vi "FOCUS_V42_H37.vi"(9 "X-pixels":sgl=256.0, 11 "Run":bool) -> (0 "Retrace pixels":sgl, 10 "Pixel Clock (Hz)":sgl)   [LabVIEW 2010] (continued)
            n1850 = Unbundle(w3125) -> ("z-positionstart (um)"=w3187:sgl, "x-positionstart (um)"=w3186:sgl, "y-positionstart (um)"=w3185:sgl, "x-positionstop (um)"=w3184:sgl, "y-positionstop (um)"=w3183:sgl, "z-positionstop (um)"=w3182:sgl, "X-pixels FreeLine"=w3181:sgl, "Y-lines FreeLine"=w3180:sgl, "Pixel Clock (Hz) FreeLine"=w3179:sgl, "Amplitude Factor"=w3171:sgl, "Pixel Clock z (Hz) FreeLine"=w3172:sgl, "phase shift [°]"=w3173:sgl, "Mode selector"=w3156:u16, "Cusp Delay"=w3159:sgl, "Fiberscope\nMode"=w3151:bool, "Pixel Clock (Hz) FScope"=w3149:sgl, "scans to read"=w3148:sgl, "LS X/Y"=w3150:bool, "DataOffset"=w3152:i32, "DataLength"=w3153:i32, "ScanLineLength"=w3154:i32, "ZSinLength"=w3155:i32)
            n1851 = call "ReScaleUDLFOCUS.vi"("ScanLineUDL"=w3146, "x jog"=w3131, "y jog"=w3130, "Rotation"=w3129, "Zoom"=w3128) -> ("ScanLineUDL"=w3145:sgl[][])
            n1852 = Index Array(array=w3145, index (col)=0 ("index (row)")) -> (element=w3178:sgl[])  [unwired: 1 in]
            n1853 = Index Array(array=w3145, index (col)=1 ("index (row)")) -> (element=w3177:sgl[])  [unwired: 1 in]
            n1854 = Bundle("ScanLineUDL"=w3178, "ScanLineUDL"=w3177) -> (w3176:T23)  [unwired: 1 in]
            n1855 = local write "z-positionstart (um)"(w3187) -> ()
            n1856 = local write "x-positionstart (um)"(w3186) -> ()
            n1857 = local write "y-positionstart (um)"(w3185) -> ()
            n1858 = local write "x-positionstop (um)"(w3184) -> ()
            n1859 = local write "y-positionstop (um)"(w3183) -> ()
            n1860 = local write "z-positionstop (um)"(w3182) -> ()
            n1861 = local write "X-pixels FreeLine"(w3181) -> ()
            n1862 = local write "Y-lines FreeLine"(w3180) -> ()
            n1863 = local write "Pixel Clock (Hz) FreeLine"(w3179) -> ()
            n1864 = local write "Amplitude Factor"(w3171) -> ()
            n1865 = local write "Pixel Clock z (Hz) FreeLine"(w3172) -> ()
            n1866 = local write "phase shift [°]"(w3173) -> ()
            n1867 = local write "Mode selector"(w3156) -> ()
            n1868 = local write "Cusp Delay"(w3159) -> ()
            n1869 = local write "Fiberscope\nMode"(w3151) -> ()
            n1870 = local write "Pixel Clock (Hz) FScope"(w3149) -> ()
            n1871 = local write "scans to read"(w3148) -> ()
            n1872 = local write "LS X/Y"(w3150) -> ()
            n1873 = local write "DataOffset"(w3152) -> ()
            n1874 = local write "DataLength"(w3153) -> ()
            n1875 = local write "ScanLineLength"(w3154) -> ()
            n1876 = local write "ZSinLength"(w3155) -> ()
            n1877 = Build Array(w3176) -> (w3175:T24)
            n1878 = local write "XY Graph 1"(w3175) -> ()
            n1879 = local write "XY Graph 2"(w3175) -> ()
            n1880 = local write "Mode selectorFScope"(w3156) -> ()
          }
        }
      }
      frame True {
        w3217 = sgl 1000000.0 ("y")
        w3261 = u8 0 ("Disabled")
        w3283 = 2
        # "Disable & grey/ hide controls"
        n1881 = local read "pixel dwell time [us] FreeLine"() -> (w3206:sgl)
        n1882 = local read "Number of stacks"() -> (w3247:sgl)
        n1883 = local read "Y-lines FreeLine"() -> (w3219:sgl)
        n1884 = local read "pixel dwell time [us]"() -> (w3207:sgl)
        n1885 = local read "frame/line indicator"() -> (w3275:u16)
        n1886 = local read "Number of frames"() -> (w3253:sgl)
        n1887 = local read "X-pixels FreeLine"() -> (w3216:sgl)
        n1888 = Multiply(x=20.0, y=w3216) -> (x*y=w3259:dbl)
        n1889 = Equal?(x=4.0 ("y"), y=w3275) -> (x = y?=w3202:bool)
        n1890 = local read "Y-lines"() -> (w3248:sgl)
        n1891 = local write "IntDevUsed"(FALSE ("IntDevUsed")) -> ()
        n1892 = Multiply(x=w3219, y=w3216) -> (x*y=w3218:sgl)
        n1893 = Greater?(x=w3247, y=sgl 1.0) -> (0:w3245:bool)
        n1894 = Initialize Array(0.0 ("element"), w3259, 3 ("dimension size")) -> (w3262:dbl[][])
        n1895 = property on="Scan format" class="Ring (strict)"("Disabled"=w3283) -> ()  [unwired: 2 in, 2 out]
        n1896 = property on="X-pixels" class="DigNum (strict)"("Disabled"=w3283) -> ()  [unwired: 2 in, 2 out]
        n1897 = property on="Y-lines" class="DigNum (strict)"("Disabled"=w3283) -> ()  [unwired: 2 in, 2 out]
        n1898 = property on="line scan time (ms)" class="DigNum (strict)"("Disabled"=w3283) -> ()  [unwired: 2 in, 2 out]
        n1899 = property on="Measurement cursor\ncheck box" class="Bool (strict)"("Disabled"=w3283) -> ()  [unwired: 2 in, 2 out]
        n1900 = property on="View line check box" class="Bool (strict)"("Disabled"=w3283) -> ()  [unwired: 2 in, 2 out]
        n1901 = property on="Zoom" class="Slide (strict)"("Disabled"=w3261) -> ()  [unwired: 2 in, 2 out]
        n1902 = property on="Rotation" class="Knob (strict)"("Disabled"=w3261) -> ()  [unwired: 2 in, 2 out]
        n1903 = local write "Ready?"(FALSE ("Ready?")) -> ()
        n1904 = Divide(x="Scanner dead time", y=w3206) -> (x/y=w3210:sgl)
        n1905 = local write "XScale"(TRUE ("XScale")) -> ()
        n1906 = property on="RUN button" class="Bool (strict)"("Visible"=FALSE) -> ()  [unwired: 2 in, 2 out]
        n1907 = Greater?(x=w3218, y=w3217) -> (0:w3221:bool)
        n1908 = Divide(x=w3217, y=w3216) -> (x/y=w3215:sgl)
        n1909 = local read "X-pixels"() -> (w3251:sgl)
        n1910 = Or(x=w3202, y=w3200) -> (x .or. y?=w3201:bool)
        n1911 = local read "Mode selectorFScope"() -> (w3239:u16)
        n1912 = case shown="True" w3245 {
          selector: w3245 -> [_ w3296]
          frame False {
          }
          frame True {
            n1913 = local write "Autosave"(w3296) -> ()
          }
        }
        n1914 = Divide(x="Scanner dead time", y=w3207) -> (x/y=w3213:sgl)
        n1915 = Select(t=w3215, s=w3221, f=w3219) -> (s? t:f=w3220:sgl)
        n1916 = local read "Fiberscope\nMode"() -> (w3240:bool)
        n1917 = Add(x=sgl 2.0, y=w3210) -> (x+y=w3209:sgl)
        n1918 = local read "Mode selector"() -> (w3284:u16)
        n1919 = local read "total x pixels"() -> (w3274:sgl)
        n1920 = local read "Intensity"() -> (w3203:sgl)
        n1921 = case shown="False" w3201 {
          tunnel: w3280 -> [w6792 w6794]
          tunnel: [w6790 w6795] -> w3279
          tunnel: w3278 -> [w6793 w6795]
          tunnel: [w6791 w6794] -> w3277
          frame False {
            n1922 = call <vilib>:"DAQmx Start Task.vi"("task/channels in"=w6793, "error in"=w6792) -> ("task out"=w6790:refnum<k21>, "error out"=w6791:errorcluster)  [unwired: 12 in]
          }
          frame True {
          }
        }
        n1923 = Multiply(x=w3248, y=w3253) -> (x*y=w3252:sgl)
        n1924 = Add(x=sgl 2.0, y=w3213) -> (x+y=w3212:sgl)
        n1925 = Round To Nearest(number=w3209) -> (nearest integer value=w3205:sgl)
        n1926 = Initialize Array(u8 0 ("element"), w3251, w3248) -> (w3285:u8[][])
        n1927 = Initialize Array(u8 0 ("element"), w3216, w3220) -> (w3281:u8[][])
        n1928 = Round To Nearest(number=w3212) -> (nearest integer value=w3204:sgl)
        n1929 = while {
          tunnel: w3294 -> [w3441]
          tunnel: w3293 -> [w3440]
          tunnel: w3292 -> [w3439]
          tunnel: [w3438] -> w3291
          tunnel: [w3437] -> w3290
          tunnel: [w3436] -> w3289
          tunnel: [w3386] -> w3288
          tunnel: [w3393] -> w3287
          tunnel: [w3435] -> w3286
          tunnel: w3285 -> [w3434]
          tunnel: w3284 -> [w3433]
          tunnel: w3281 -> [w3432]
          tunnel: w3279 -> [w3431]
          tunnel: w3277 -> [w3430]
          tunnel: w3274 -> [w3429]
          tunnel: [w3428] -> w3272
          tunnel: [w3427] -> w3271
          tunnel: [w3425] -> w3269
          tunnel: w3267 -> [w3424]
          tunnel: w3266 -> [w3423]
          tunnel: w3262 -> [w3419]
          tunnel: w3216 -> [w3418]
          tunnel: w3243 -> [w3406]
          tunnel: w3244 -> [w3405]
          tunnel: w3258 -> [w3408]
          tunnel: w3257 -> [w3407]
          tunnel: [w3383] -> w3256
          tunnel: [w3397] -> w3255
          tunnel: w3242 -> [w3381]
          tunnel: w3241 -> [w3380]
          tunnel: w3254 -> [w3417]
          tunnel: w3252 -> [w3416]
          tunnel: w3251 -> [w3415]
          tunnel: [w3414] -> w3250
          tunnel: [w3413] -> w3249
          tunnel: w3248 -> [w3412]
          tunnel: w3220 -> [w3411]
          tunnel: w3240 -> [w3373]
          tunnel: w3239 -> [w3372]
          tunnel: w3238 -> [w3371]
          tunnel: w3237 -> [w3370]
          tunnel: w3236 -> [w3369]
          tunnel: w3235 -> [w3368]
          tunnel: w3234 -> [w3367]
          tunnel: [w3366] -> w3233
          tunnel: [w3365] -> w3232
          tunnel: w3231 -> [w3364]
          tunnel: [w3351] -> w3230
          tunnel: w3229 -> [w3341]
          tunnel: w3228 -> [w3340]
          tunnel: [w3339] -> w3227
          tunnel: [w3336] -> w3226
          tunnel: [w3332] -> w3225
          tunnel: [w3331] -> w3224
          tunnel: w3223 -> [w3330]
          tunnel: w3222 -> [w3329]
          tunnel: w3204 -> [w3308]
          tunnel: w3205 -> [w3307]
          tunnel: w3203 -> [w3305]
          tunnel: w3200 -> [w3298]
          i -> [w3402]
          stop <- w3399 stop-if-true
          n1930 = local read "Trigger?"() -> (w3376:bool)
          n1931 = local write "Intensity"(w3305) -> ()
          n1932 = flat-sequence {
            tunnel: w3405 -> [w6664]
            tunnel: w3406 -> [w6663]
            tunnel: [w6662] -> w3303
            tunnel: [w6661] -> w3304
            frame #0 {
              n1933 = call <vilib>:"DAQmx Start Task.vi"("task/channels in"=w6664, "error in"=w6663) -> ("task out"=w6661:refnum<k21>, "error out"=w6662:errorcluster)  [unwired: 12 in]
            }
          }
          n1934 = property class="DAQmx Write"(reference=w3304, error in=w3303) -> ("Status:Total Samples Per Channel Generated"=w3302:dbl)  [unwired: 2 out]
          n1935 = case shown="True" w3376 {
            tunnel: w3408 -> [w6630 w6639]
            tunnel: w3407 -> [w6629 w6638]
            tunnel: [w6628 w6636] -> w3389
            tunnel: [w6627 w6637] -> w3388
            tunnel: w3303 -> [w6624 w6633]
            tunnel: w3304 -> [w6625 w6635]
            tunnel: [w6625 w6634] -> w3375
            tunnel: [w6624 w6632] -> w3374
            tunnel: w3302 -> [_ w6631]
            frame False {
              w6626 = TRUE ("data")
              # "open shutter before\ngathering data"
              n1936 = call-poly <vilib>:"DAQmx Write (Digital Bool 1Line 1Point).vi"("task/channels in"=w6630, "data"=w6626, "error in"=w6629) -> ("task out"=w6627:refnum<k21>, "error out"=w6628:errorcluster)  [unwired: 10 in, 1 out]
              "Shutter open" <- w6626
            }
            frame True {
              n1937 = while {
                tunnel: w6639 -> [w6653]
                tunnel: w6638 -> [w6652]
                tunnel: [w6651] -> w6637
                tunnel: [w6647] -> w6636
                tunnel: w6635 -> [w6650]
                tunnel: [w6649] -> w6634
                tunnel: w6633 -> [w6648]
                tunnel: [w6646] -> w6632
                tunnel: w6631 -> [w6640]
                stop <- w6643 stop-if-true
                n1938 = property class="DAQmx Write"(reference=w6650, error in=w6648) -> (reference out=w6649:refnum<k21>, error out=w6646:errorcluster, "Status:Total Samples Per Channel Generated"=w6641:dbl)
                n1939 = Unbundle By Name(w6646) -> ("status"=w6644:bool)
                n1940 = Not Equal?(x=w6641, y=w6640) -> (x != y?=w6642:bool)
                n1941 = case shown="True" w6642 {
                  tunnel: w6653 -> [w6655 w6659]
                  tunnel: w6652 -> [w6654 w6658]
                  tunnel: [w6655 w6657] -> w6651
                  tunnel: [w6654 w6656] -> w6647
                  frame False {
                  }
                  frame True {
                    w6660 = TRUE ("data")
                    n1942 = local write "Shutter open"(w6660) -> ()
                    n1943 = call-poly <vilib>:"DAQmx Write (Digital Bool 1Line 1Point).vi"("task/channels in"=w6659, "data"=w6660, "error in"=w6658) -> ("task out"=w6657:refnum<k21>, "error out"=w6656:errorcluster)  [unwired: 10 in, 1 out]
                  }
                }
                n1944 = Unbundle By Name(w6647) -> ("status"=w6645:bool)
                n1945 = Compound Arithmetic op=OR(w6642, w6645, w6644) -> (w6643:bool)
              }
            }
          }
          n1946 = local read "Pixel Clock (Hz) FScope"() -> (w3360:sgl)
          n1947 = Initialize Array(u8 0 ("element"), 768 ("dimension size")) -> (w3309:u8[])
          n1948 = local read "Scan mode"() -> (w3306:u16)
          n1949 = local write "Save?"(FALSE ("Save?")) -> ()
          n1950 = Reciprocal(x=w3360) -> (1/x=w3359:sgl)
          n1951 = local read "frame/line indicator"() -> (w3410:u16)
          n1952 = local read "ScanLineFreeLine"() -> (w3321:sgl[][])
          n1953 = Decrement(x="Number of stacks") -> (x-1=w3403:sgl)
          n1954 = flat-sequence {
            tunnel: w3426 -> [w6767]
            tunnel: [w6767] -> w3425
            tunnel: w3352 -> [_]
            tunnel: w3333 -> [_]
            tunnel: [w6729] -> w3323
            frame #0 {
              w6741 = "filename000000"  # name
              n1955 = local read "Pixel Clock z (Hz) FreeLine"() -> (w6738:sgl)
              n1956 = local read "Pixel Clock (Hz) FreeLine"() -> (w6757:sgl)
              n1957 = local read "Pixel Clock (Hz) FScope"() -> (w6732:sgl)
              n1958 = local read "x-positionstart (um)"() -> (w6765:sgl)
              n1959 = local read "y-positionstart (um)"() -> (w6764:sgl)
              n1960 = local read "z-positionstart (um)"() -> (w6766:sgl)
              n1961 = local read "x-positionstop (um)"() -> (w6763:sgl)
              n1962 = local read "y-positionstop (um)"() -> (w6761:sgl)
              n1963 = local read "z-positionstop (um)"() -> (w6762:sgl)
              n1964 = local read "ScanLineLength"() -> (w6754:i32)
              n1965 = local read "X-pixels FreeLine"() -> (w6759:sgl)
              n1966 = local read "Amplitude Factor"() -> (w6737:sgl)
              n1967 = local read "Fiberscope\nMode"() -> (w6733:bool)
              n1968 = local read "Y-lines FreeLine"() -> (w6758:sgl)
              n1969 = local read "DataLength"() -> (w6755:i32)
              n1970 = local read "DataOffset"() -> (w6740:i32)
              n1971 = local read "phase shift [°]"() -> (w6739:sgl)
              n1972 = local read "ZSinLength"() -> (w6753:i32)
              n1973 = local read "Mode selector"() -> (w6756:u16)
              n1974 = local read "scans to read"() -> (w6731:sgl)
              n1975 = local read "Cusp Delay"() -> (w6736:sgl)
              n1976 = local read "LS X/Y"() -> (w6730:bool)
              n1977 = Bundle("z-positionstart (um)"=w6766, "x-positionstart (um)"=w6765, "y-positionstart (um)"=w6764, "x-positionstop (um)"=w6763, "y-positionstop (um)"=w6761, "z-positionstop (um)"=w6762, "X-pixels FreeLine"=w6759, "Y-lines FreeLine"=w6758, "Pixel Clock (Hz) FreeLine"=w6757, "Amplitude Factor"=w6737, "Pixel Clock z (Hz) FreeLine"=w6738, "phase shift [°]"=w6739, "Mode selector"=w6756, "Cusp Delay"=w6736, "Fiberscope\nMode"=w6733, "Pixel Clock (Hz) FScope"=w6732, "scans to read"=w6731, "LS X/Y"=w6730, "DataOffset"=w6740, "DataLength"=w6755, "ScanLineLength"=w6754, "ZSinLength"=w6753) -> (w6760:T22)  [unwired: 1 in]
              n1978 = local read "ScanSignals"() -> (w6744:dbl[][])
              n1979 = Index Array(array=w6744, index (col)=0 ("disabled index (col)")) -> (element=w6747:dbl[])  [unwired: 1 in]
              n1980 = Index Array(array=w6744, index (col)=1 ("disabled index (col)")) -> (element=w6752:dbl[])  [unwired: 1 in]
              n1981 = local read "Retrace pixels"() -> (w6775:sgl)
              n1982 = local read "line scan time (ms)"() -> (w6776:sgl)
              n1983 = Array Max & Min(array=w6747) -> (max value=w6748:dbl, min value=w6749:dbl)  [unwired: 2 out]
              n1984 = local read "Scan Block Length"() -> (w6782:sgl)
              n1985 = local read "Number of frames"() -> (w6778:sgl)
              n1986 = Array Max & Min(array=w6752) -> (max value=w6750:dbl, min value=w6751:dbl)  [unwired: 2 out]
              n1987 = local read "Number of stacks"() -> (w6735:sgl)
              n1988 = local read "Program Version"() -> (w6789:u16)
              n1989 = local read "Time interval [s]"() -> (w6734:sgl)
              n1990 = local read "Pixel Clock (Hz)"() -> (w6781:sgl)
              n1991 = local read "IntDevUsed"() -> (w6784:bool)
              n1992 = local read "x-step (um)"() -> (w6773:sgl)
              n1993 = local read "y-step (um)"() -> (w6772:sgl)
              n1994 = local read "z-step (um)"() -> (w6774:sgl)
              n1995 = Subtract(x=w6748, y=w6749) -> (x-y=w6743:dbl)
              n1996 = Subtract(x=w6750, y=w6751) -> (x-y=w6742:dbl)
              n1997 = local read "Averaging"() -> (w6777:u16)
              n1998 = local read "Intensity"() -> (w6783:sgl)
              n1999 = local read "Rotation"() -> (w6769:sgl)
              n2000 = local read "X-pixels"() -> (w6780:sgl)
              n2001 = local read "Y-lines"() -> (w6779:sgl)
              n2002 = local read "Zoom"() -> (w6768:sgl)
              n2003 = local read "x jog"() -> (w6771:sgl)
              n2004 = local read "y jog"() -> (w6770:sgl)
              n2005 = local read "Date"() -> (w6787:string)
              n2006 = local read "start"() -> (w6786:u32)
              n2007 = local read "Time"() -> (w6788:string)
              n2008 = local read "stop"() -> (w6785:u32)
              n2009 = Bundle("Program Version"=w6789, "name"=w6741, "Time"=w6788, "Date"=w6787, "start"=w6786, "stop"=w6785, "IntDevUsed"=w6784, "Intensity"=w6783, "Scan Block Length"=w6782, "Pixel Clock (Hz)"=w6781, "X-pixels"=w6780, "Y-lines"=w6779, "Number of frames"=w6778, "Averaging"=w6777, "line scan time (ms)"=w6776, "Retrace pixels"=w6775, "z-step (um)"=w6774, "x-step (um)"=w6773, "y-step (um)"=w6772, w6743, w6742, "x jog"=w6771, "y jog"=w6770, "Rotation"=w6769, "Zoom"=w6768, "Number of stacks"=w6735, "Time interval [s]"=w6734, w6760) -> (w6728:T21)  [unwired: 1 in]
              n2010 = call "HeadertestFOCUS.vi"("HeaderCluster"=w6728) -> ("Header"=w6729:u8[])
              "Header" <- w6729
            }
          }
          n2011 = Equal?(x=w3410, y=u16 1) -> (x = y?=w3400:bool)
          n2012 = local read "Parameters"() -> (w3382:T2)
          n2013 = case shown="False" w3373 {
            tunnel: w3441 -> [w3517 w6050]
            tunnel: w3440 -> [w3516 w6049]
            tunnel: w3439 -> [w3515 w6048]
            tunnel: [w3514 w6022] -> w3438
            tunnel: [w3513 w6023] -> w3437
            tunnel: [w3512 w6024] -> w3436
            tunnel: [w3511 w6027] -> w3435
            tunnel: w3434 -> [w3510 w6019]
            tunnel: w3433 -> [w3509 _]
            tunnel: w3432 -> [w3508 _]
            tunnel: w3431 -> [w3507 w6039]
            tunnel: w3430 -> [w3506 w6038]
            tunnel: w3429 -> [w3505 _]
            tunnel: [w3504 w6020] -> w3428
            tunnel: [w3503 w6021] -> w3427
            tunnel: [w3502 w6028] -> w3426
            tunnel: w3424 -> [w3501 w6043]
            tunnel: w3423 -> [w3500 w6042]
            tunnel: [w3499 w6029] -> w3422
            tunnel: [w3498 w6030] -> w3421
            tunnel: [w3497 w6031] -> w3420
            tunnel: w3419 -> [w3496 _]
            tunnel: w3418 -> [w3495 _]
            tunnel: w3417 -> [w3494 w6037]
            tunnel: w3416 -> [w3493 _]
            tunnel: w3415 -> [w3492 w6010]
            tunnel: [w3491 w6035] -> w3414
            tunnel: [w3490 w6034] -> w3413
            tunnel: w3412 -> [w3489 w6006]
            tunnel: w3411 -> [w3488 _]
            tunnel: [w3487 w6036] -> w3343
            tunnel: [w3486 w6033] -> w3396
            tunnel: [w3485 w6032] -> w3395
            tunnel: [w3484 w6026] -> w3394
            tunnel: w3389 -> [w3483 w6040]
            tunnel: w3388 -> [w3482 w6041]
            tunnel: [w3481 w6025] -> w3387
            tunnel: w3382 -> [w3480 _]
            tunnel: w3381 -> [w3479 w6047]
            tunnel: w3380 -> [w3478 w6046]
            tunnel: [w3477 w6009] -> w3377
            tunnel: w3375 -> [w3476 w6045]
            tunnel: w3374 -> [w3475 w6044]
            tunnel: w3372 -> [_ w6051]
            tunnel: w3371 -> [_ w6018]
            tunnel: w3370 -> [_ w6017]
            tunnel: w3369 -> [_ w6016]
            tunnel: w3368 -> [w3473 w6015]
            tunnel: w3367 -> [w3474 w6014]
            tunnel: [w3473 w6013] -> w3366
            tunnel: [w3474 w6012] -> w3365
            tunnel: w3359 -> [_ w6007]
            tunnel: [w3472 w6002] -> w3339
            tunnel: [w3471 w6001] -> w3336
            tunnel: w3341 -> [w3470 _]
            tunnel: w3340 -> [w3469 _]
            tunnel: [w3468 w6000] -> w3332
            tunnel: [w3467 w5999] -> w3331
            tunnel: w3330 -> [w3466 w6000]
            tunnel: w3329 -> [w3465 w5999]
            tunnel: w3309 -> [w3464 _]
            tunnel: w3308 -> [w3463 _]
            tunnel: w3307 -> [w3462 _]
            tunnel: w3306 -> [w3461 _]
            tunnel: w3298 -> [w3460 _]
            tunnel: "Channel selector" -> [w3459 _]
            frame False {
              n2014 = case shown="0, Default" w3509 {
                tunnel: w3475 -> [w3617 w4234 w4719 w5022 w5261 w5724]
                tunnel: w3476 -> [w3640 w4235 w4743 w5023 w5260 w5726]
                tunnel: w3517 -> [w3639 w4242 w4740 w5031 w5297 w5796]
                tunnel: w3516 -> [w3638 w4243 w4741 w5030 w5298 w5795]
                tunnel: w3515 -> [w3637 w4244 w4742 w5029 w5299 w5794]
                tunnel: [w3636 w4242 w4740 w5031 w5297 w5796] -> w3514
                tunnel: [w3635 w4243 w4741 w5030 w5298 w5795] -> w3513
                tunnel: [w3634 w4244 w4742 w5029 w5299 w5794] -> w3512
                tunnel: [w3628 w4233 w4743 w5021 w5262 w5725] -> w3481
                tunnel: [w3618 w4232 w4719 w5020 w5271 w5723] -> w3484
                tunnel: [w3629 w4247 w4737 w5026 w5265 w5791] -> w3511
                tunnel: [w3613 w4238 w4731 w5009 w5264 w5787] -> w3502
                tunnel: w3501 -> [w3633 w4246 w4738 w5027 w5301 w5792]
                tunnel: w3500 -> [w3616 w4241 w4734 w5012 w5288 w5786]
                tunnel: w3510 -> [w3631 w4220 _ _ w5300 _]
                tunnel: w3505 -> [w3632 w4245 w4739 _ w5290 _]
                tunnel: w3508 -> [_ _ _ w5028 _ w5793]
                tunnel: w3495 -> [_ _ _ w4989 _ w5749]
                tunnel: w3507 -> [w3604 w4217 w4736 w5024 w5281 w5789]
                tunnel: w3506 -> [w3603 w4216 w4720 w4987 w5280 w5760]
                tunnel: [w3601 w4214 w4720 w4987 w5278 w5760] -> w3490
                tunnel: [w3602 w4215 w4736 w5024 w5279 w5789] -> w3491
                tunnel: w3479 -> [w3577 w4228 w4723 w5016 w5263 w5782]
                tunnel: w3478 -> [w3576 w4226 w4722 w5015 w5258 w5781]
                tunnel: [w3577 w4227 w4723 w5014 w5263 w5779] -> w3504
                tunnel: [w3576 w4225 w4722 w5013 w5258 w5780] -> w3503
                tunnel: [_ 0 ("DataLength") 0 ("DataLength") 0 ("DataLength") 0 ("DataLength") _] -> w3499
                tunnel: [_ 0 ("DataLength") 0 ("DataLength") 0 ("DataLength") 0 ("DataLength") _] -> w3498
                tunnel: [_ 768 ("DataLength") 768 ("DataLength") 768 ("DataLength") 768 ("DataLength") 768 ("DataLength")] -> w3497
                tunnel: w3496 -> [_ _ _ w5003 _ w5775]
                tunnel: w3482 -> [w3612 w4224 w4727 w4993 w5277 w5765]
                tunnel: w3483 -> [w3611 w4223 w4726 w4992 w5276 w5764]
                tunnel: [w3610 w4213 w4725 w4991 w5275 w5762] -> w3486
                tunnel: [w3609 w4222 w4724 w4990 w5274 w5763] -> w3485
                tunnel: w3494 -> [w3591 w4177 w4709 w4985 w5250 w5756]
                tunnel: [w3589 w4221 w4709 w4985 w5250 w5756] -> w3487
                tunnel: w3493 -> [_ w4218 w4714 _ w5273 _]
                tunnel: w3492 -> [_ w4219 w4713 _ w5272 _]
                tunnel: w3489 -> [w3545 _ _ _ _ _]
                tunnel: w3488 -> [_ _ _ _ _ w5735]
                tunnel: w3480 -> [w3579 _ _ _ _ _]
                tunnel: [_ w4212 w4721 w4988 w5259 w5761] -> w3477
                tunnel: [w3562 w4207 w4711 w4981 w5252 w5755] -> w3472
                tunnel: [w3561 w4206 w4710 w4980 w5251 w5754] -> w3471
                tunnel: w3470 -> [_ _ _ w4981 _ w5755]
                tunnel: w3469 -> [_ _ _ w4980 _ w5754]
                tunnel: [w3560 w4205 w4708 w4979 w5249 w5752] -> w3468
                tunnel: [w3559 w4204 w4707 w4978 w5248 w5753] -> w3467
                tunnel: w3466 -> [w3560 w4205 w4708 _ w5249 _]
                tunnel: w3465 -> [w3559 w4204 w4707 _ w5248 _]
                tunnel: w3464 -> [w3526 w4190 w4693 w4963 w5234 w5731]
                tunnel: w3463 -> [w3553 w4189 w4692 _ w5233 _]
                tunnel: w3462 -> [_ _ _ w4962 _ w5712]
                tunnel: w3461 -> [w3552 w4178 w4691 _ w5232 _]
                tunnel: w3460 -> [w3538 _ _ _ _ _]
                tunnel: w3459 -> [w3523 w4169 w4690 w4961 w5229 w5711]
                frame 0, Default {
                  w3581 = FALSE ("button 1")
                  n2015 = local read "Position piezo [µm]"() -> (w3549:sgl)
                  n2016 = property on="Property Node" class="VI"() -> ("VI Path"=w3531:path)  [unwired: 2 in, 2 out]
                  n2017 = local read "[µm] per pixel at zoom 1"() -> (w3546:sgl)
                  n2018 = Strip Path(path=w3531) -> (stripped path=w3532:path)  [unwired: 1 out]
                  n2019 = flat-sequence {
                    tunnel: w3616 -> [w3649]
                    tunnel: [w3649] -> w3615
                    frame #0 {
                      n2020 = Tick Count (ms)() -> (millisecond timer value=w3650:u32)
                      n2021 = local write "Parameters"(T2."Offset Rotation" ("Parameters")) -> ()
                      n2022 = local write "start"(w3650) -> ()
                    }
                  }
                  n2023 = local read "scattering length [µm]"() -> (w3540:sgl)
                  n2024 = case shown="True" "FocusModeSelector" {
                    tunnel: [w3641 w3647] -> w3619
                    tunnel: [w3642 w3646] -> w3578
                    frame True {
                      n2025 = local read "Scan Block Length"() -> (w3642:sgl)
                      n2026 = Multiply(x=w3642, y=u32 1) -> (x*y=w3643:sgl)
                      n2027 = To Long Integer(number=w3643) -> (32bit integer=w3641:i32)
                    }
                    frame False {
                      n2028 = local read "Scan Block Length"() -> (w3646:sgl)
                      n2029 = To Long Integer(number=0 ("y")) -> (32bit integer=w3647:i32)
                    }
                  }
                  n2030 = property class="VI"() -> ("Front Panel Window:Window Bounds"=w3572:T25)  [unwired: 2 in, 2 out]
                  n2031 = local write "Focus"(FALSE ("Focus")) -> ()
                  n2032 = Build Path(base path=w3532, name or relative path="Stack.tmp") -> (appended path=w3533:path)
                  n2033 = local read "Zoom"() -> (w3580:sgl)
                  n2034 = local read "Rotation z"() -> (w3548:sgl)
                  n2035 = local read "Intensity"() -> (w3541:sgl)
                  n2036 = local read "total y pixels"() -> (w3570:sgl)
                  n2037 = Divide(x=w3549, y=sgl 40.0) -> (x/y=w3547:sgl)
                  n2038 = local read "x jog"() -> (w3621:sgl)
                  n2039 = local read "y jog"() -> (w3620:sgl)
                  n2040 = call <vilib>:"Open_Create_Replace File.vi"("advisory dialog? (display:T)"=FALSE, "function (open:0)"=T8."create or replace", "file path"=w3533) -> ("error out"=w3537:errorcluster, "refnum"=w3536:refnum<file>)  [unwired: 5 in, 2 out]
                  n2041 = local read "z-positionstart (um)"() -> (w3590:sgl)
                  n2042 = call <vilib>:"Initialize Mouse.vi"() -> ("error out"=w3587:errorcluster, "device ID"=w3588:refnum<k1>)  [unwired: 10 in]
                  n2043 = call <vilib>:"Intialize Keyboard.vi"() -> ("error out"=w3557:errorcluster, "device ID"=w3558:refnum<k1>)  [unwired: 10 in]
                  n2044 = local read "On?"() -> (w3543:bool)
                  n2045 = local read "Intensity"() -> (w3574:sgl)
                  n2046 = local read "GetFirst"() -> (w3564:bool)
                  n2047 = local read "GetLast"() -> (w3565:bool)
                  n2048 = Divide(x=w3570, y=u32 3) -> (x/y=w3568:sgl)
                  n2049 = Set File Position(refnum=w3536, from (0:start)=enum16{"start", "end", "current"}."start" ("pos mode (rel. to end:1)"), error in=w3537) -> (refnum out=w3520:refnum<file>, error out=w3519:errorcluster)  [unwired: 1 in]
                  n2050 = Write to Binary File(file (use dialog)=w3520, data=w3526, error in=w3519, 5:FALSE ("prepend array or string size? (T)")) -> (refnum out=w3528:refnum<file>, error out=w3527:errorcluster)  [unwired: 2 in, 1 out]
                  n2051 = Greater Or Equal?(x=w3523, y=u16 3) -> (x >= y?=w3521:bool)
                  n2052 = Not(x=w3543) -> (.not. x?=w3542:bool)
                  n2053 = Bundle(sgl 64.0, sgl 64.0, sgl 1.0, "Zoom"=w3580, "x jog"=w3621, "y jog"=w3620, sgl 0.0, sgl 1.0, "Rotation z"=w3548, w3547, "[µm] per pixel at zoom 1"=w3546, "Intensity"=w3541, "scattering length [µm]"=w3540) -> (w3623:T26)  [unwired: 1 in]
                  n2054 = To Word Integer(number=w3568) -> (16bit integer=w3567:i16)
                  n2055 = Tick Count (ms)() -> (millisecond timer value=w3630:u32)
                  n2056 = while {
                    tunnel: [w3715] -> w3629
                    tunnel: [w3713] -> w3614
                    tunnel: w3633 -> [w3785]
                    tunnel: w3615 -> [w3784]
                    shift-right: [w3808] -> w3562
                    shift-left: w3631 -> [w3771]
                    tunnel: w3632 -> [w3788]
                    tunnel: w3639 -> [w3815]
                    tunnel: w3638 -> [w3816]
                    tunnel: w3637 -> [w3739]
                    tunnel: w3617 -> [w3744]
                    tunnel: [w3815] -> w3636
                    tunnel: [w3816] -> w3635
                    tunnel: [w3739] -> w3634
                    tunnel: [w3741] -> w3618
                    shift-right: [w3807] -> w3561
                    shift-left: w3631 -> [w3778]
                    shift-right: [w3809] -> _
                    shift-left: w3630 -> [w3795]
                    shift-right: [w3758] -> w3622
                    shift-left: w3623 -> [w3789]
                    shift-right: [w3748] -> _
                    shift-left: w3619 -> [w3805]
                    shift-right: [w3804] -> _
                    shift-left: w3578 -> [w3802]
                    shift-right: [w3800] -> _
                    shift-left: i16 0 -> [w3726]
                    shift-right: [w3728] -> _
                    shift-left: w3574 -> [w3791]
                    shift-right: [w3806] -> w3628
                    shift-left: w3640 -> [w3745]
                    tunnel: w3612 -> [w3786]
                    tunnel: w3611 -> [w3743]
                    tunnel: [w3786] -> w3610
                    tunnel: [w3743] -> w3609
                    tunnel: w3604 -> [w3777]
                    tunnel: w3603 -> [w3776]
                    tunnel: [w3775] -> w3602
                    tunnel: [w3742] -> w3601
                    tunnel: w3591 -> [w3770]
                    shift-right: [w3767] -> _
                    shift-left: w3590 -> [w3768]
                    tunnel: [w3769] -> w3589
                    tunnel: w3588 -> [w3765]
                    tunnel: w3587 -> [w3764]
                    tunnel: [w3740] -> w3586
                    tunnel: [w3766] -> w3585
                    shift-right: [w3757] -> _
                    shift-left: 0 ("y") -> [w3760]
                    shift-right: [w3755] -> _
                    shift-left: w3581 -> [w3756]
                    shift-right: [w3753] -> _
                    shift-left: 0 ("y") -> [w3754]
                    shift-right: [w3751] -> _
                    shift-left: w3581 -> [w3752]
                    tunnel: [w3728] -> w3575
                    tunnel: w3572 -> [w3727]
                    shift-right: [w3725] -> _
                    shift-left: w3567 -> [w3724]
                    shift-right: [w3721] -> _
                    shift-left: w3565 -> [w3719]
                    shift-right: [w3722] -> _
                    shift-left: w3564 -> [w3720]
                    shift-right: [w3718] -> _
                    shift-left: FALSE ("GetLast") -> [w3717]
                    tunnel: w3558 -> [w3711]
                    tunnel: w3557 -> [w3710]
                    tunnel: [w3709] -> w3555
                    tunnel: [w3708] -> w3554
                    tunnel: w3553 -> [w3704]
                    tunnel: w3552 -> [w3700]
                    tunnel: w3545 -> [w3693]
                    shift-right: [w3681] -> _
                    shift-left: w3542 -> [w3690]
                    shift-right: [w3686] -> _
                    shift-left: i16 0 ("0, 1") -> [w3687]
                    tunnel: "FocusModeSelector" -> [w3677]
                    tunnel: w3538 -> [w3672]
                    tunnel: w3523 -> [_]
                    shift-right: [w3660] -> w3525
                    shift-left: w3528 -> [w3663]
                    shift-right: [w3659] -> w3524
                    shift-left: w3527 -> [w3662]
                    tunnel: w3521 -> [_]
                    i -> [w3699]
                    stop <- w3731 stop-if-true
                    # "Focus mode"
                    # "DIO Read reads one\nline of data at a time"
                    n2057 = local read "total x pixels"() -> (w3801:sgl)
                    n2058 = local read "Scan Cut-Off (either end)"() -> (w3787:sgl)
                    n2059 = local read "total y pixels"() -> (w3798:sgl)
                    n2060 = local read "IntensityScaleMax"() -> (w3705:sgl)
                    n2061 = local read "Scan Block Length"() -> (w3703:sgl)
                    n2062 = call "ResetToZeroFOCUS.vi"("UpperLimit"=w3798, "Running Index"=w3805) -> ("New Index"=w3749:i32)
                    n2063 = Equal To 0?(x=w3699) -> (x = 0?=w3750:bool)
                    n2064 = case shown="True" w3750 {
                      tunnel: w3788 -> [w4032 w4037]
                      tunnel: [w4032 w4036] -> w3783
                      tunnel: w3787 -> [w4031 w4035]
                      tunnel: [w4031 w4034] -> w3773
                      tunnel: w3704 -> [_ w4033]
                      frame False {
                      }
                      frame True {
                        n2065 = Add(x=w4037, y=w4033) -> (x+y=w4036:sgl)
                        n2066 = Add(x=w4035, y=w4033) -> (x+y=w4034:sgl)
                      }
                    }
                    n2067 = call-poly <vilib>:"DAQmx Read (Digital 1D U32 1Chan NSamp).vi"("task/channels in"=w3785, "number of samples per channel"=w3783, "error in"=w3784) -> ("task out"=w3716:refnum<k21>, "data"=w3702:u32[], "error out"=w3714:errorcluster)  [unwired: 10 in]
                    n2068 = call "OffsetControlFOCUS.vi"("Offset Control"="Offset Control", "Scan Parameters"=w3789) -> ("Scan Parameters"=w3794:T27)
                    n2069 = Increment(x=w3749) -> (x+1=w3748:i32)
                    n2070 = call "keyboardAcquireFOCUS.vi"("device ID"=w3711, "error in (no error)"=w3710) -> ("device ID"=w3709:refnum<k1>, "Up?"=w3707:bool, "Zero?"=w3683:bool, "Down?"=w3706:bool, "error out"=w3708:errorcluster)  [unwired: 13 in]
                    n2071 = Multiply(x=w3801, y=w3703) -> (x*y=w3793:sgl)
                    n2072 = Divide(x="Position piezo [µm]", y=sgl 40.0) -> (x/y=w3694:sgl)
                    n2073 = local read "X-pixels"() -> (w3782:sgl)
                    n2074 = Not(x=w3672) -> (.not. x?=w3674:bool)
                    n2075 = In Range and Coerce(upper limit=sgl 0.0, x="Intensity", lower limit=w3705) -> (coerced(x)=w3728:sgl)  [unwired: 1 out]
                    n2076 = case shown="1" w3700 {
                      tunnel: w3699 -> [_ w3935]
                      tunnel: w3702 -> [w3930 w3933]
                      tunnel: [w3930 w3932] -> w3701
                      frame 0, Default {
                      }
                      frame 1 {
                        n2077 = call "testoddevenFOCUS.vi"("Numeric"=w3935) -> ("Boolean"=w3934:bool)
                        n2078 = case shown="True" w3934 {
                          tunnel: w3933 -> [w3937 w3941]
                          tunnel: [w3936 w3938] -> w3932
                          tunnel: "Shift" -> [_ w3940]
                          frame False {
                            n2079 = Reverse 1D Array(array=w3937) -> (reversed array=w3936:u32[])
                          }
                          frame True {
                            n2080 = Round Toward -Infinity(1:w3940) -> (0:w3939:sgl)
                            n2081 = Rotate 1D Array(1:w3941, 2:w3939) -> (0:w3938:u32[])
                          }
                        }
                      }
                    }
                    n2082 = Multiply(x="[µm] per pixel at zoom 1", y=w3693) -> (x*y=w3691:sgl)
                    n2083 = Multiply(x=w3749, y=w3801) -> (x*y=w3747:sgl)
                    n2084 = Add(x="Cusp Delay", y=w3773) -> (x+y=w3774:sgl)
                    n2085 = event shown="[0] Timeout" {
                      selector: _ -> [_ _ _ _]
                      dyn-events: _ -> [_ _ _ _]
                      timeout: 0 -> [_ _ _ _]
                      event Timeout {
                        n2086 = event-data() -> ()  [unwired: 1 in, 2 out]
                      }
                      event "Zero": Mouse Down {
                        n2087 = event-data() -> ()  [unwired: 1 in, 1 out]
                        n2088 = local write "Rotation"(sgl 0.0 ("Rotation")) -> ()
                      }
                      event "Zoom 1": Mouse Down {
                        n2089 = event-data() -> ()  [unwired: 1 in, 1 out]
                        n2090 = local write "Zoom"(sgl 1.0 ("Zoom")) -> ()
                      }
                      event "Reset": Mouse Down {
                        n2091 = event-data() -> ()  [unwired: 1 in, 1 out]
                        n2092 = local write "Rotation"(sgl 0.0 ("Rotation")) -> ()
                        n2093 = local write "Zoom"(sgl 1.0 ("Zoom")) -> ()
                      }
                    }
                    n2094 = Multiply(x="Rotation", y=sgl -1.0) -> (x*y=w3780:sgl)
                    n2095 = local write "Intensity"(w3728) -> ()
                    n2096 = Boolean To (0,1)(Boolean=w3683) -> (0, 1=w3686:i16)
                    n2097 = Array Subset "Extract DI0"(array=w3701, index=w3774, length=w3782) -> (w3746:u32[])
                    n2098 = Subtract(x=w3747, y=w3793) -> ()  [unwired: 1 out]
                    n2099 = Subtract(x=w3780, y=sgl 360.0) -> (x-y=w3697:sgl)
                    n2100 = local read "Channel selector"() -> (w3656:u8)
                    n2101 = case shown="False" w3707 {
                      tunnel: "Intensity" -> [w3946 w3950]
                      tunnel: w3706 -> [_ w3949]
                      tunnel: w3705 -> [w3942 w3948]
                      frame True {
                        n2102 = Add(x=w3946, y=sgl 0.0001) -> (x+y=w3944:sgl)
                        n2103 = In Range and Coerce(upper limit=sgl 0.0, x=w3944, lower limit=w3942) -> (coerced(x)=w3943:sgl)  [unwired: 1 out]
                        n2104 = local write "Intensity"(w3943) -> ()
                      }
                      frame False {
                        n2105 = case shown="True" w3949 {
                          tunnel: w3950 -> [_ w3955]
                          tunnel: w3948 -> [_ w3951]
                          frame False {
                          }
                          frame True {
                            n2106 = Subtract(x=w3955, y=sgl 0.0001) -> (x-y=w3953:sgl)
                            n2107 = In Range and Coerce(upper limit=sgl 0.0, x=w3953, lower limit=w3951) -> (coerced(x)=w3952:sgl)  [unwired: 1 out]
                            n2108 = local write "Intensity"(w3952) -> ()
                          }
                        }
                      }
                    }
                    n2109 = Not Equal?(x=w3728, y=w3791) -> (x != y?=w3676:bool)
                    n2110 = Subtract(x=w3687, y=w3686) -> (x-y=w3685:i16)
                    n2111 = Split Number(x=w3746) -> (hi(x)=w3671:u16[], lo(x)=w3670:u16[])
                    n2112 = And(x=w3676, y=w3674) -> (x .and. y?=w3675:bool)
                    n2113 = Equal?(x=w3685, y=i16 1 ("0, 1")) -> (x = y?=w3682:bool)
                    n2114 = case shown="0, Default" w3656 {
                      tunnel: w3671 -> [w3847 w3852 w3857 w3862 w3867 w3872]
                      tunnel: [w3846 w3851 w3854 w3861 w3866 w3869] -> w3669
                      tunnel: [w3844 w3849 w3856 w3859 w3864 w3871] -> w3668
                      tunnel: w3670 -> [w3845 w3850 w3855 w3860 w3865 w3870]
                      tunnel: [w3843 w3848 w3853 w3858 w3863 w3868] -> w3667
                      frame 0, Default {
                        n2115 = Split Number(x=w3847) -> (hi(x)=w3846:u8[], lo(x)=w3844:u8[])
                        n2116 = Split Number(x=w3845) -> (lo(x)=w3843:u8[])  [unwired: 1 out]
                      }
                      frame 1 {
                        n2117 = Split Number(x=w3852) -> (hi(x)=w3851:u8[], lo(x)=w3848:u8[])
                        n2118 = Split Number(x=w3850) -> (lo(x)=w3849:u8[])  [unwired: 1 out]
                      }
                      frame 2 {
                        n2119 = Split Number(x=w3857) -> (hi(x)=w3853:u8[], lo(x)=w3856:u8[])
                        n2120 = Split Number(x=w3855) -> (lo(x)=w3854:u8[])  [unwired: 1 out]
                      }
                      frame 3 {
                        n2121 = Split Number(x=w3862) -> (hi(x)=w3861:u8[], lo(x)=w3859:u8[])
                        n2122 = Split Number(x=w3860) -> (lo(x)=w3858:u8[])  [unwired: 1 out]
                      }
                      frame 4 {
                        n2123 = Split Number(x=w3867) -> (hi(x)=w3866:u8[], lo(x)=w3863:u8[])
                        n2124 = Split Number(x=w3865) -> (lo(x)=w3864:u8[])  [unwired: 1 out]
                      }
                      frame 5 {
                        n2125 = Split Number(x=w3872) -> (hi(x)=w3868:u8[], lo(x)=w3871:u8[])
                        n2126 = Split Number(x=w3870) -> (lo(x)=w3869:u8[])  [unwired: 1 out]
                      }
                    }
                    n2127 = Decrement(x=w3703) -> (x-1=w3797:sgl)
                    n2128 = case shown="True" w3675 {
                      tunnel: w3728 -> [_ w4025]
                      tunnel: w3777 -> [w4024 w4029]
                      tunnel: w3776 -> [w4023 w4028]
                      tunnel: [w4024 w4027] -> w3775
                      tunnel: [w4023 w4026] -> w3742
                      frame False {
                      }
                      frame True {
                        n2129 = Build Array(sgl 0.0 ("element"), w4025) -> ()  [unwired: 1 out]
                        n2130 = call-poly <vilib>:"DAQmx Write (Analog DBL 1Chan 1Samp).vi"("task/channels in"=w4029, "data"=w4025, "error in"=w4028) -> ("task out"=w4027:refnum<k21>, "error out"=w4026:errorcluster)  [unwired: 10 in, 1 out]
                      }
                    }
                    n2131 = Greater Or Equal?(x=w3656, y=u16 3) -> (x >= y?=w3655:bool)
                    n2132 = Greater Or Equal?(x=w3802, y=w3797) -> (x >= y?=w3803:bool)
                    n2133 = case shown="True" w3682 {
                      tunnel: w3690 -> [w3875 w3877]
                      tunnel: [w3875 w3876] -> w3681
                      frame False {
                      }
                      frame True {
                        n2134 = Not(x=w3877) -> (.not. x?=w3876:bool)
                      }
                    }
                    n2135 = case shown="True" w3681 {
                      tunnel: "Rotation z" -> [w3873 _]
                      tunnel: [w3873 sgl 0.0 ("Rotation z")] -> w3688
                      frame False {
                      }
                      frame True {
                      }
                    }
                    n2136 = Bundle(cluster=w3794, "X Pixels"=w3801, "Y Lines"=w3798, "Actual Line"=w3747, "Zoom"="Zoom", "Rotation Angle (deg)"=w3697, "Lines to Generate"=w3793, "Rotation z"=w3688, "Position piezo"=w3694, "z scaling"=w3691, "Intensity"="Intensity", "Scattering length (um)"="scattering length [µm]") -> (w3759:T27)  [unwired: 2 in]
                    n2137 = Tick Count (ms)() -> (millisecond timer value=w3796:u32)
                    n2138 = local read "total y pixels"() -> (w3799:sgl)
                    n2139 = property class="DAQmx Read"(reference=w3716, error in=w3714) -> (reference out=w3715:refnum<k21>, error out=w3713:errorcluster, "Status:Available Samples Per Channel"=w3712:u32)
                    n2140 = case shown="True" w3803 {
                      tunnel: w3745 -> [w4052 w4083]
                      tunnel: w3744 -> [w4051 w4080]
                      tunnel: [w4052 w4082] -> w3806
                      tunnel: [w4051 w4081] -> w3741
                      tunnel: w3802 -> [w4050 _]
                      tunnel: [w4049 u32 0 ("y")] -> w3804
                      tunnel: [w4048 w4077] -> w3766
                      tunnel: w3765 -> [w4048 w4076]
                      tunnel: w3764 -> [w4047 w4075]
                      tunnel: [w4047 w4074] -> w3740
                      tunnel: [0 w4072] -> w3762
                      tunnel: w3760 -> [w4044 w4070]
                      tunnel: w3759 -> [w4045 w4056]
                      tunnel: [w4045 w4069] -> w3758
                      tunnel: [w4044 w4059] -> w3757
                      tunnel: w3756 -> [w4043 w4068]
                      tunnel: [w4043 w4067] -> w3755
                      tunnel: w3754 -> [w4042 w4066]
                      tunnel: [w4042 w4057] -> w3753
                      tunnel: w3752 -> [w4041 w4061]
                      tunnel: [w4041 w4060] -> w3751
                      tunnel: w3727 -> [_ w4058]
                      tunnel: w3677 -> [_ w4053]
                      frame False {
                        n2141 = Increment(x=w4050) -> (x+1=w4049:sgl)
                      }
                      frame True {
                        n2142 = local read "OriginalScanSignals"() -> (w4055:dbl[][])
                        n2143 = call "mouseAcquireFOCUS.vi"("device ID"=w4076, "error in (no error)"=w4075) -> ("device ID"=w4077:refnum<k1>, "axis info"=w4073:T28, "button info"=w4071:T29, "error out"=w4074:errorcluster)  [unwired: 14 in]
                        n2144 = Unbundle(w4073) -> ("Horizontal"=w4059:i32, "Vertical"=w4057:i32, "Scrolling"=w4072:i32)
                        n2145 = call "rotationzoomFOCUS.vi"("Focus mode"=w4053, "scan signals"=w4055, "Scan Parameters"=w4056) -> ("scan signals"=w4054:dbl[][], "Rotation Matrix"=w4064:dbl[][])
                        n2146 = call "withinplotareaFOCUS.vi"("Front Panel Window:Window Bounds"=w4058, "Cursor:Y"=w4057, "Cursor:X"=w4059) -> ("within Plot?"=w4065:bool)
                        n2147 = case shown="True" w4065 {
                          tunnel: w4071 -> [_ w4104]
                          tunnel: w4070 -> [_ w4091]
                          tunnel: [w4087 w4102] -> w4069
                          tunnel: w4068 -> [w4088 w4100]
                          tunnel: [w4088 w4097] -> w4067
                          tunnel: w4056 -> [w4087 w4099]
                          tunnel: w4066 -> [_ w4090]
                          tunnel: w4059 -> [_ w4092]
                          tunnel: w4057 -> [_ w4089]
                          tunnel: w4064 -> [_ w4096]
                          tunnel: w4061 -> [w4086 w4095]
                          tunnel: [w4086 w4093] -> w4060
                          frame False {
                          }
                          frame True {
                            n2148 = Unbundle(w4104) -> ("button 1"=w4097:bool, "button 2"=w4093:bool)  [unwired: 2 out]
                            n2149 = Subtract(x=w4090, y=w4089) -> (x-y=w4098:i32)
                            n2150 = And(x=w4095, y=w4093) -> (x .and. y?=w4094:bool)
                            n2151 = Subtract(x=w4091, y=w4092) -> (x-y=w4103:i32)
                            n2152 = And(x=w4100, y=w4097) -> (x .and. y?=w4101:bool)
                            n2153 = case shown="True" w4101 {
                              tunnel: w4099 -> [w4105 w4134]
                              tunnel: w4103 -> [w4107 w4123]
                              tunnel: [w4105 w4126] -> w4102
                              tunnel: w4098 -> [w4106 w4121]
                              tunnel: w4096 -> [_ w4119]
                              tunnel: w4094 -> [w4108 _]
                              frame False {
                                n2154 = case shown="True" w4108 {
                                tunnel: w4107 -> [_ w4112]
                                tunnel: w4106 -> [_ w4111]
                                frame False {
                                }
                                frame True {
                                n2155 = local read "Rotation"() -> (w4110:sgl)
                                n2156 = call "MouseRotate.vi"("Rotation"=w4110, "Delta Y"=w4111, "Delta X"=w4112) -> ("Rotation"=w4109:sgl)
                                n2157 = local write "Rotation"(w4109) -> ()
                                }
                                }
                              }
                              frame True {
                                n2158 = Unbundle(w4134) -> ("X Pixels"=w4132:sgl, "Y Lines"=w4131:sgl, "Actual Line"=w4130:sgl, "Zoom"=w4118:sgl, "X Offset"=w4133:sgl, "Y Offset"=w4125:sgl, "Rotation Angle (deg)"=w4128:sgl, "Lines to Generate"=w4127:sgl, "Rotation z"=w4117:sgl, "Position piezo"=w4116:sgl, "z scaling"=w4115:sgl, "Intensity"=w4114:sgl, "Scattering length (um)"=w4113:sgl)
                                n2159 = call "OffsetRotationFOCUS.vi"("Rotation Matrix"=w4119, "Zoom"=w4118, "Offset Y"=w4121, "Offset X"=w4123) -> ("Offset Y"=w4120:sgl, "Offset X"=w4122:sgl)
                                n2160 = Add(x=w4122, y=w4133) -> (x+y=w4129:sgl)
                                n2161 = Add(x=w4120, y=w4125) -> (x+y=w4124:sgl)
                                n2162 = Bundle("X Pixels"=w4132, "Y Lines"=w4131, "Actual Line"=w4130, "Zoom"=w4118, w4129, w4124, "Rotation Angle (deg)"=w4128, "Lines to Generate"=w4127, "Rotation z"=w4117, "Position piezo"=w4116, "z scaling"=w4115, "Intensity"=w4114, "Scattering length (um)"=w4113) -> (w4126:T30)  [unwired: 1 in]
                              }
                            }
                          }
                        }
                        n2163 = Index Array(array=w4054, index (row)=1 ("index")) -> (element=w4078:dbl[])  [unwired: 1 in]
                        n2164 = Index Array(array=w4054, index (row)=0 ("index")) -> (element=w4079:dbl[])  [unwired: 1 in]
                        n2165 = Bundle("scan signals"=w4079, "scan signals"=w4078) -> (w4084:T31)  [unwired: 1 in]
                        n2166 = local write "Galvos"(w4084) -> ()
                        n2167 = call-poly <vilib>:"DAQmx Write (Analog 2D DBL NChan NSamp).vi"("task/channels in"=w4083, "data"=w4054, "error in"=w4080) -> ("task out"=w4082:refnum<k21>, "error out"=w4081:errorcluster)  [unwired: 10 in, 1 out]
                      }
                    }
                    n2168 = Subtract(x=w3796, y=w3795) -> (x-y=w3812:u32)
                    n2169 = Decrement(x=w3799) -> (x-1=w3723:sgl)
                    n2170 = case shown="1" w3700 {
                      tunnel: w3669 -> [w3880 w3887]
                      tunnel: [w3880 w3886] -> w3666
                      tunnel: w3699 -> [_ w3889]
                      tunnel: w3668 -> [w3879 w3884]
                      tunnel: [w3879 w3883] -> w3665
                      tunnel: w3667 -> [w3878 w3882]
                      tunnel: [w3878 w3881] -> w3664
                      frame 0, Default {
                      }
                      frame 1 {
                        n2171 = local read "Shift"() -> (w3885:sgl)
                        n2172 = call "testoddevenFOCUS.vi"("Numeric"=w3889) -> ("Boolean"=w3888:bool)
                        n2173 = case shown="True" w3888 {
                          tunnel: w3887 -> [w3892 w3919]
                          tunnel: [w3892 w3921] -> w3886
                          tunnel: w3885 -> [_ w3894]
                          tunnel: w3884 -> [w3891 w3907]
                          tunnel: [w3891 w3906] -> w3883
                          tunnel: w3882 -> [w3890 w3895]
                          tunnel: [w3890 w3893] -> w3881
                          frame False {
                          }
                          frame True {
                            n2174 = Round Toward -Infinity(1:w3894) -> (0:w3911:sgl)
                            n2175 = Round Toward -Infinity(1:w3894) -> (0:w3926:sgl)
                            n2176 = Round Toward -Infinity(1:w3894) -> (0:w3902:sgl)
                            n2177 = To Word Integer(number=w3907) -> (16bit integer=w3917:i16[])
                            n2178 = To Word Integer(number=w3919) -> (16bit integer=w3918:i16[])
                            n2179 = To Word Integer(number=w3895) -> (16bit integer=w3896:i16[])
                            n2180 = Array Subset(array=w3917, index=1) -> (w3910:i16[])  [unwired: 1 in]
                            n2181 = Array Subset(array=w3918, index=1) -> (w3927:i16[])  [unwired: 1 in]
                            n2182 = Array Subset(array=w3896, index=1) -> (w3903:i16[])  [unwired: 1 in]
                            n2183 = Subtract(x=w3894, y=w3911) -> (x-y=w3912:sgl)
                            n2184 = Subtract(x=w3894, y=w3926) -> (x-y=w3925:sgl)
                            n2185 = Subtract(x=w3894, y=w3902) -> (x-y=w3901:sgl)
                            n2186 = Subtract(x=w3917, y=w3910) -> (x-y=w3914:i16[])
                            n2187 = Subtract(x=w3918, y=w3927) -> (x-y=w3923:i16[])
                            n2188 = Subtract(x=w3896, y=w3903) -> (x-y=w3899:i16[])
                            n2189 = Build Array (concatenate)(0 ("index"), w3914) -> (w3915:i32[])
                            n2190 = Build Array (concatenate)(0 ("index"), w3923) -> (w3922:i32[])
                            n2191 = Build Array (concatenate)(0 ("index"), w3899) -> (w3898:i32[])
                            n2192 = Multiply(x=w3912, y=w3915) -> (x*y=w3913:sgl[])
                            n2193 = Multiply(x=w3925, y=w3922) -> (x*y=w3924:sgl[])
                            n2194 = Multiply(x=w3901, y=w3898) -> (x*y=w3900:sgl[])
                            n2195 = Add(x=w3917, y=w3913) -> (x+y=w3908:sgl[])
                            n2196 = To Unsigned Byte Integer(number=w3908) -> (unsigned 8bit integer=w3906:u8[])
                            n2197 = Add(x=w3918, y=w3924) -> (x+y=w3929:sgl[])
